vi "Close Recordset.vi"(4 "error in":errorcluster, 7 "Recordset":refnum<k7>) -> (0 "error out":errorcluster)   [LabVIEW 2020, in "ADO Database Drivers.lvlib"]
uses:
  ADO Database Drivers.lvlib
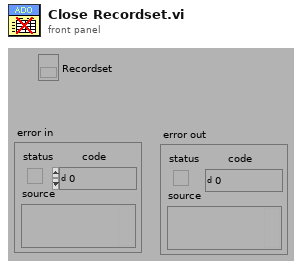
[diagram p1: front panel]
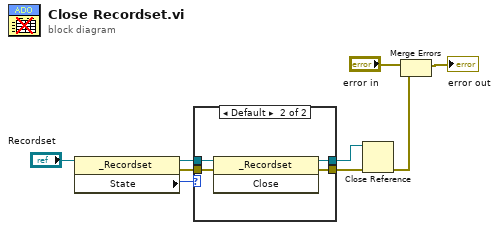
[diagram p0: block diagram]
diagram:
  n1 = property class="_Recordset"(reference="Recordset") -> (reference out=w8:refnum<k7>, error out=w6:errorcluster, "State"=w7:i32)  [unwired: 1 in]
  n2 = case shown="Default" w7 {
    tunnel: [w11 w13] -> w4
    tunnel: w8 -> [w10 w15]
    tunnel: w6 -> [w11 w14]
    tunnel: [w10 w12] -> w5
    frame 0 {
    }
    frame Default {
      n3 = invoke class="_Recordset" method="Close"(reference=w15, error in=w14) -> (reference out=w12:refnum<k7>, error out=w13:errorcluster)  [unwired: 1 in, 1 out]
    }
  }
  n4 = Close Reference(reference=w5, error in (no error)=w4) -> (error out=w1:errorcluster)
  n5 = Merge Errors("error in", w1) -> (→"error out":errorcluster)
